vi "XY_conf.vi"(4 "error in (no error)":errorcluster caption="错误输入（无错误）", 5 "方式":enum16{"写入", "读取"}(ring), 6 "产品":string, 7 "XY图引用":refnum<vi>) -> (0 "error out":errorcluster caption="错误输出")   [LabVIEW 2020]
uses:
  <vilib>/Utility/config.llb/Read Key (Double).vi
  <vilib>/Utility/config.llb/Write Key (Double).vi
  <vilib>/Utility/config.llb/NI_LVConfig.lvlib
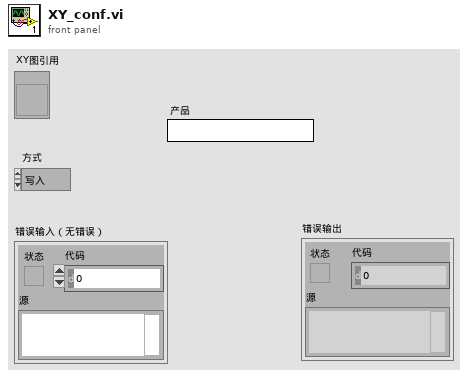
[diagram p1: front panel]
types:
  T1 = typedef "NI_LVConfig.lvlib/Config Data RefNum.ctl" = refnum<k1>
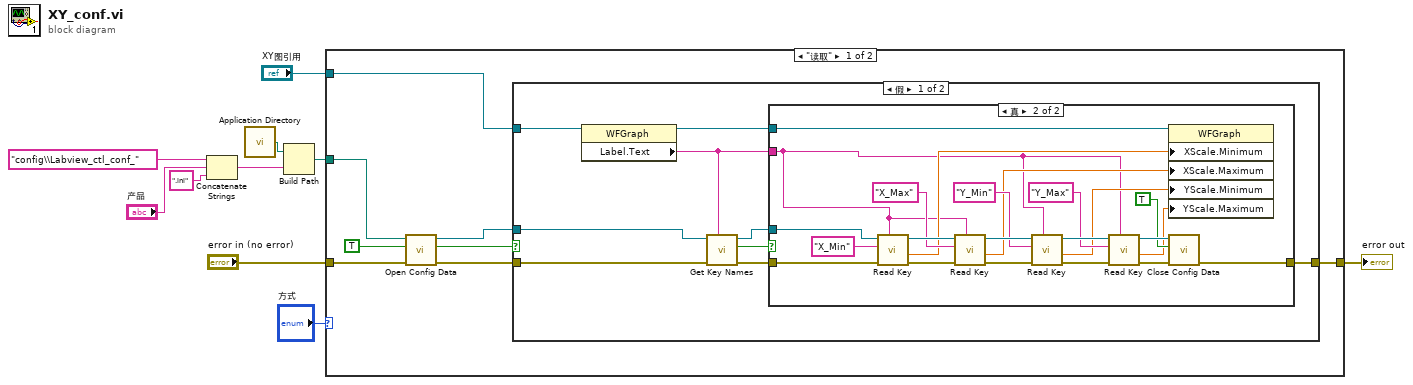
[diagram p0: block diagram]
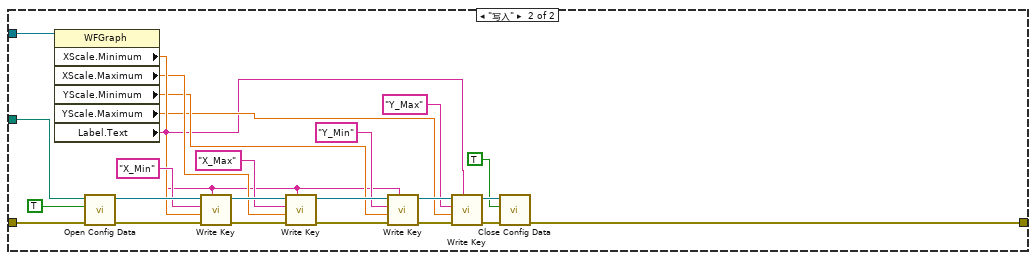
[diagram p4: hidden frame]
diagram:
  n1 = Concatenate Strings("config\\Labview_ctl_conf_" ("名称或相对路径"), "产品", ".ini" ("名称或相对路径")) -> (w1:string)
  n2 = call <vilib>:"Application Directory.vi"() -> ("Application Directory"=w5:path)
  n3 = Build Path(base path=w5, name or relative path=w1) -> (appended path=w8:path)
  n4 = case shown="\"读取\"" "方式" {
    tunnel: "XY图引用" -> [w14 w76]
    tunnel: w8 -> [w17 w74]
    tunnel: "error in (no error)" -> [w16 w71]
    tunnel: [w15 w57] -> w6
    frame "读取" {
      n5 = call <vilib>:"Open Config Data.vi"("error in (no error)"=w16, "create file if necessary (T)"=TRUE, "configuration file path"=w17) -> ("error out"=w12:errorcluster, "file created?"=w11:bool, "refnum"=w13:T1)  [unwired: 6 in]
      n6 = case shown="假" w11 {
        tunnel: [w27 w51] -> w15
        tunnel: w14 -> [w26 _]
        tunnel: w13 -> [w24 _]
        tunnel: w12 -> [w23 w51]
        frame False {
          n7 = property class="WFGraph"(reference=w26) -> (reference out=w25:refnum<vi>, "Label.Text"=w20:string)  [unwired: 1 in, 1 out]
          n8 = call <vilib>:"Get Key Names.vi"("section"=w20, "error in (no error)"=w23, "refnum"=w24) -> ("error out"=w22:errorcluster, "section exists?"=w19:bool, "refnum out"=w21:T1)  [unwired: 5 in, 1 out]
          n9 = case shown="真" w19 {
            tunnel: [w28 w38] -> w27
            tunnel: w25 -> [_ w36]
            tunnel: w22 -> [w28 w31]
            tunnel: w21 -> [_ w30]
            tunnel: w20 -> [_ w29]
            frame False {
            }
            frame True {
              n10 = call-poly <vilib>:"Read Key.vi"("section"=w29, "error in (no error)"=w31, "key"="X_Min", "refnum"=w30) -> ("error out"=w42:errorcluster, "value"=w35:dbl, "refnum out"=w49:T1)  [unwired: 4 in, 1 out]
              n11 = call-poly <vilib>:"Read Key.vi"("section"=w29, "error in (no error)"=w42, "key"="X_Max", "refnum"=w49) -> ("error out"=w41:errorcluster, "value"=w34:dbl, "refnum out"=w48:T1)  [unwired: 4 in, 1 out]
              n12 = call-poly <vilib>:"Read Key.vi"("section"=w29, "error in (no error)"=w41, "key"="Y_Min", "refnum"=w48) -> ("error out"=w40:errorcluster, "value"=w33:dbl, "refnum out"=w47:T1)  [unwired: 4 in, 1 out]
              n13 = call-poly <vilib>:"Read Key.vi"("section"=w29, "error in (no error)"=w40, "key"="Y_Max", "refnum"=w47) -> ("error out"=w39:errorcluster, "value"=w32:dbl, "refnum out"=w46:T1)  [unwired: 4 in, 1 out]
              n14 = property class="WFGraph"(reference=w36, "XScale.Minimum"=w35, "XScale.Maximum"=w34, "YScale.Minimum"=w33, "YScale.Maximum"=w32) -> ()  [unwired: 1 in, 2 out]
              n15 = call <vilib>:"Close Config Data.vi"("error in (no error)"=w39, "write file if changed (T)"=TRUE, "refnum"=w46) -> ("error out"=w38:errorcluster)  [unwired: 7 in, 1 out]
            }
          }
        }
        frame True {
        }
      }
    }
    frame "写入" {
      n16 = property class="WFGraph"(reference=w76) -> ("XScale.Minimum"=w69:dbl, "XScale.Maximum"=w56:dbl, "YScale.Minimum"=w55:dbl, "YScale.Maximum"=w54:dbl, "Label.Text"=w53:string)  [unwired: 1 in, 2 out]
      n17 = call <vilib>:"Open Config Data.vi"("error in (no error)"=w71, "create file if necessary (T)"=TRUE, "configuration file path"=w74) -> ("error out"=w72:errorcluster, "refnum"=w73:T1)  [unwired: 6 in, 1 out]
      n18 = call-poly <vilib>:"Write Key.vi"("section"=w53, "error in (no error)"=w72, "value"=w69, "key"="X_Min", "refnum"=w73) -> ("error out"=w61:errorcluster, "refnum out"=w68:T1)  [unwired: 4 in, 1 out]
      n19 = call-poly <vilib>:"Write Key.vi"("section"=w53, "error in (no error)"=w61, "value"=w56, "key"="X_Max", "refnum"=w68) -> ("error out"=w60:errorcluster, "refnum out"=w67:T1)  [unwired: 4 in, 1 out]
      n20 = call-poly <vilib>:"Write Key.vi"("section"=w53, "error in (no error)"=w60, "value"=w55, "key"="Y_Min", "refnum"=w67) -> ("error out"=w59:errorcluster, "refnum out"=w66:T1)  [unwired: 4 in, 1 out]
      n21 = call-poly <vilib>:"Write Key.vi"("section"=w53, "error in (no error)"=w59, "value"=w54, "key"="Y_Max", "refnum"=w66) -> ("error out"=w58:errorcluster, "refnum out"=w65:T1)  [unwired: 4 in, 1 out]
      n22 = call <vilib>:"Close Config Data.vi"("error in (no error)"=w58, "write file if changed (T)"=TRUE, "refnum"=w65) -> ("error out"=w57:errorcluster)  [unwired: 7 in, 1 out]
    }
  }
  "error out" <- w6
